vi "Begin-End Map.vi"(8 "Error In":errorcluster) -> (0 "Error Out":errorcluster)   [LabVIEW 2017, in "Tests.lvlib" / "Reader.lvlib"]
uses:
  Reader.lvlib
  src/LabPack/Public/Reader/Private/Begin Map by Value.vi
  src/LabPack/Public/Reader/Private/End Map by Value.vi
  <vilib>/addons/_JKI Toolkits/Caraya/classes/Test/Test.lvclass
  <vilib>/addons/_JKI Toolkits/Caraya/classes/Assert/Assert.lvclass
  src/LabPack/Public/Reader/Reader.lvclass
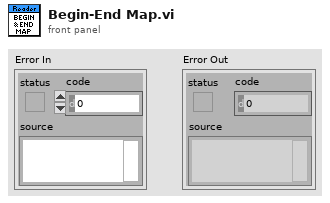
[diagram p1: front panel]
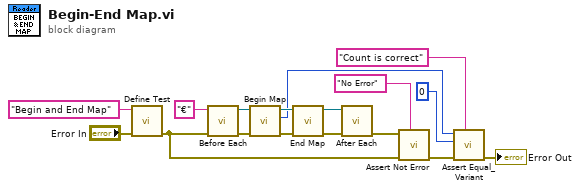
[diagram p0: block diagram]
diagram:
  n1 = call <vilib>:"Define Test.vi"("error in (no error)"="Error In", "Label (VI Title)"="Begin and End Map") -> ("error out"=w7:errorcluster)  [unwired: 9 in]
  n2 = call "Before Each.vi"("Error In"=w7, "Data"="€") -> ("Error Out"=w15:errorcluster, "Reader"=w14:refnum<class "Reader.lvclass">)  [unwired: 8 in]
  n3 = call-poly "Begin Map.vi"("Error In"=w15, "Reader In"=w14) -> ("Error Out"=w12:errorcluster, "Count"=w3:u32, "Reader Out"=w13:refnum<class "Reader.lvclass">)  [unwired: 7 in]
  n4 = call-poly "End Map.vi"("Error In"=w12, "Reader In"=w13) -> ("Error Out"=w10:errorcluster, "Reader Out"=w11:refnum<class "Reader.lvclass">)  [unwired: 8 in]
  n5 = call "After Each.vi"("Error In"=w10, "Reader In"=w11) -> ("Error Out"=w9:errorcluster)  [unwired: 9 in]
  n6 = call <vilib>:"Assert Not Error.vi"("Label"="No Error", "error in (no error)"=w7, "Not Error?"=w9) -> ("error out"=w6:errorcluster)  [unwired: 8 in]
  n7 = call <vilib>:"Assert Equal_Variant.vi"("Label"="Count is correct", "error in (no error)"=w6, "Y"=u32 0 ("Count"), "X"=w3) -> ("error out"=→"Error Out":errorcluster)  [unwired: 7 in]
